vi "Const_SQLMapper.vi"() -> (0 "SQLMapper":refnum<class "SqlMapper.lvclass">)   [LabVIEW 2020, in "ORM_Dapper.lvlib"]
uses:
  ORM_Dapper.lvlib
  <vilib>/Viviota/shared/ORM.lvlibp/ORM/SqlMapper/SqlMapper.lvclass
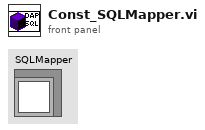
[diagram p1: front panel]
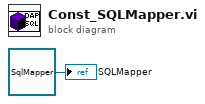
[diagram p0: block diagram]
diagram:
  "SQLMapper" <- refnum<class "SqlMapper.lvclass"> refnum ("SQLMapper")
